vi "QPlus_Analyzer 3.0.vi"() -> ()   [LabVIEW 2017]
uses:
  <vilib>/express/express shared/transition.llb/Dynamic To Waveform Array.vi
  <vilib>/express/express signal manip/GetorSetDDTAttributes/Set DDT Attributes/SetT0.vi
  <vilib>/express/express shared/transition.llb/Waveform Array To Dynamic.vi
  <vilib>/express/express signal manip/GetorSetDDTAttributes/Set DDT Attributes/Set DDT Properties.xnode
  <instrlib>/Stanford Research 830/Stanford Research 830.lvlib
  <instrlib>/Agilent 3352X Series/Agilent 3352X Series.lvlib
panel:
  out "Resonance Frequency":dbl
  out "Y Signal":cluster{"Y":dbl[], "Y":dbl[]}[](graph)
  out "X Signal":cluster{"Y":dbl[], "Y":dbl[]}[](graph)
  in  "Reference name":refnum<visa-resource-name>
  in  "VISA resource name":refnum<visa-resource-name>
  in  "Sensitivity (26: 1 V/uA)":i8(ring)=20 items=["Auto Gain"=-1, "2 nV/fA"=0, "5 nV/fA"=1, "10 nV/fA"=2, "20 nV/fA"=3, "50 nV/fA"=4, "100 nV/fA"=5, "200 nV/fA"=6, "500 nV/fA"=7, "1 uV/pA"=8, "2 uV/pA"=9, "5 uV/pA"=10, "10 uV/pA"=11, "20 uV/pA"=12, "50 uV/pA"=13, "100 uV/pA"=14, "200 uV/pA"=15, "500 uV/pA"=16, "1 mV/nA"=17, "2 mV/nA"=18, "5 mV/nA"=19, "10 mV/nA"=20, "20 mV/nA"=21, "50 mV/nA"=22, "100 mV/nA"=23, "200 mV/nA"=24, "500 mV/mA"=25, "1 V/uA"=26]
  in  "Time Constant (6: 10ms)":u16(ring)=6 items=["10 us", "30 us", "100 us", "300 us", "1 ms", "3 ms", "10 ms", "30 ms", "100 ms", "300 ms", "1 s", "3 s", "10 s", "30 s", "100 s", "300 s", "1 ks", "3 ks", "10 ks", "30 ks"]
  in  "Save File Name":path=path "C:/Users/transport/Desktop/qPlus Tip Test/Data" caption="Filename"
  in  "Time Between Points (sec)":dbl=0.05 format="%#_1f"
  in  "Sine Output Amplitude (1 V)":dbl=0.1
  in  "Starting Frequency (Hz)":dbl=29000.0
  in  "Final Frequency (Hz)":dbl=32000.0
  in  "Step Size (Hz)":dbl=10.0
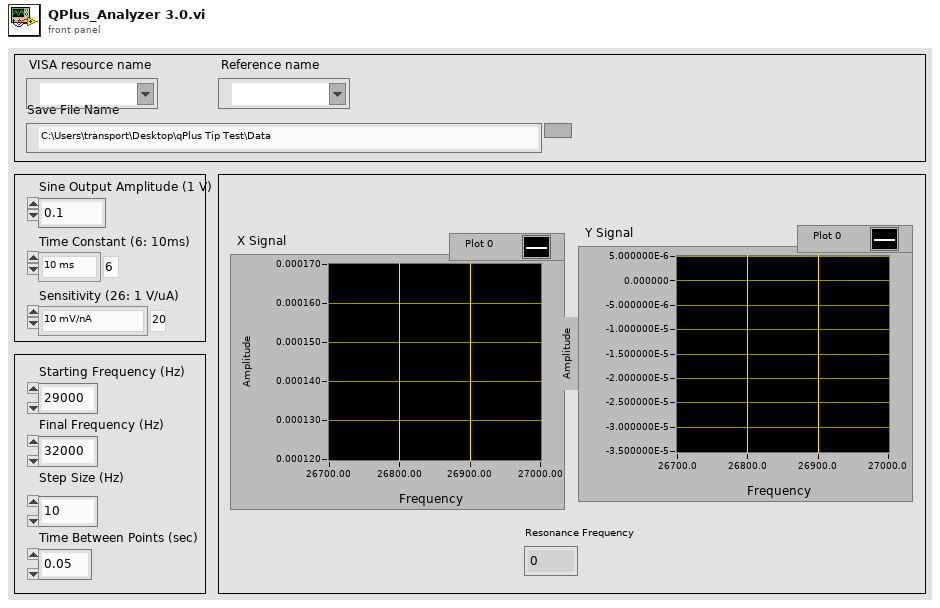
[diagram p1: front panel]
types:
  T1 = cluster{"X-Value":dbl, "Y-Value":dbl, "R-Value":dbl, "Theta-Value":dbl, "Aux In 1 Value":dbl, "Aux In 2 Value":dbl, "Aux In 3 Value":dbl, "Aux In 4 Value":dbl, "Reference Frequency":dbl, "Channel 1 Display":dbl, "Channel 2 Display":dbl}
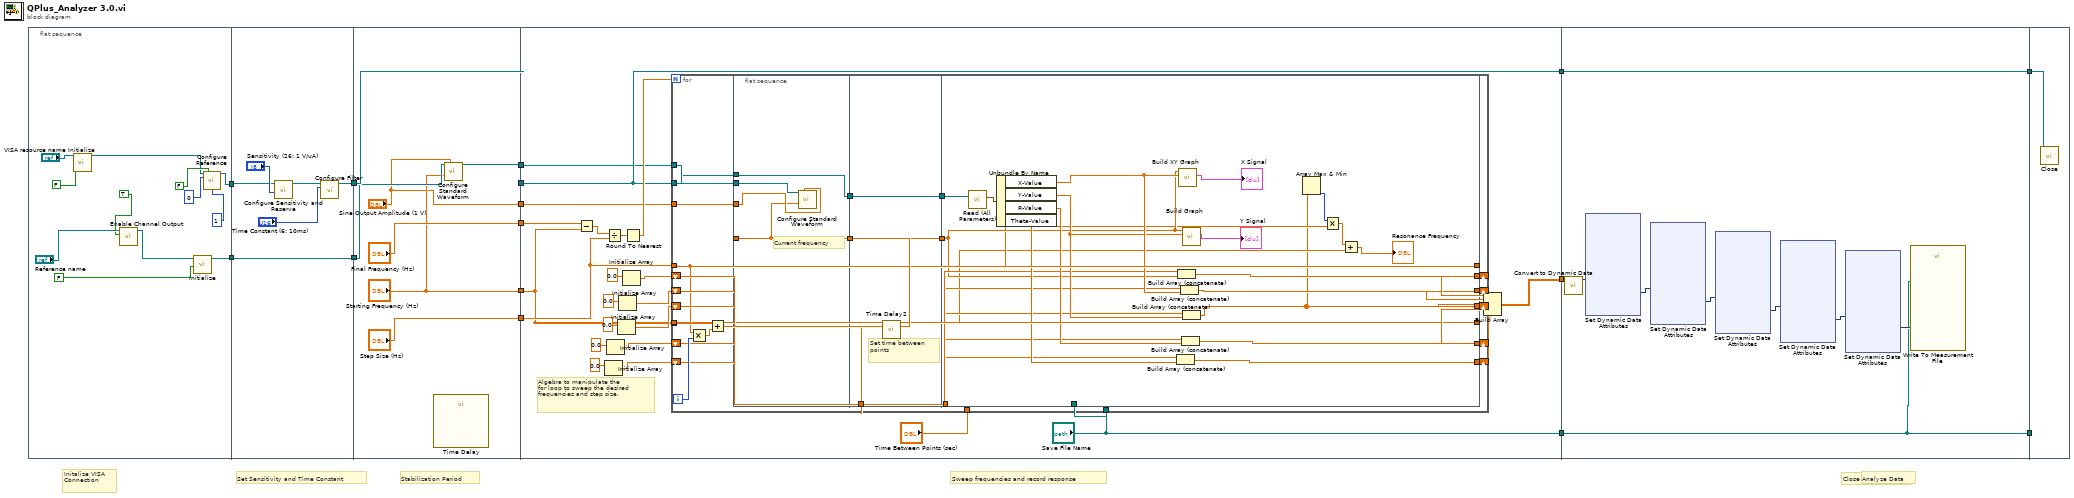
[diagram p0: block diagram]
diagram:
  # "Stabilization Period"
  # "Analyze Data"
  # "Close connection"
  # "Sweep frequencies and record response"
  # "Set Sensitivity and Time Constant"
  # "Initalize VISA\nConnection"
  n1 = flat-sequence {
    tunnel: [w23] -> w15
    tunnel: [w24] -> w7
    tunnel: [w30] -> w14
    tunnel: w15 -> [w29]
    tunnel: [w28] -> w8
    tunnel: w7 -> [w28]
    tunnel: w14 -> [w38]
    tunnel: [w38] -> w13
    tunnel: ["Starting Frequency (Hz)"] -> w12
    tunnel: ["Final Frequency (Hz)"] -> w11
    tunnel: ["Step Size (Hz)"] -> w10
    tunnel: ["Sine Output Amplitude (1 V)"] -> w9
    tunnel: w8 -> [w36]
    tunnel: [w37] -> w6
    tunnel: w13 -> [w64]
    tunnel: [w64] -> w5
    tunnel: ["Save File Name"] -> w3
    tunnel: w12 -> [w41]
    tunnel: w11 -> [w62]
    tunnel: w10 -> [w61]
    tunnel: w9 -> [w60]
    tunnel: w6 -> [w59]
    tunnel: [w42] -> w1
    tunnel: w5 -> [w132]
    tunnel: [w132] -> w4
    tunnel: w3 -> [w124]
    tunnel: [w124] -> w2
    tunnel: w1 -> [w125]
    tunnel: w4 -> [w203]
    tunnel: w2 -> [_]
    frame #0 {
      n2 = call <instrlib>:"Initialize.vi"("Reset (True)"=FALSE, "VISA resource name"="VISA resource name") -> ("VISA resource name out"=w16:refnum<visa-resource-name>)  [unwired: 8 in, 1 out]
      n3 = call <instrlib>:"Enable Channel Output.vi"("Enable Output (T: Enable)"=TRUE, "VISA resource name"="Reference name") -> ("VISA resource name out"=w18:refnum<visa-resource-name>)  [unwired: 8 in, 1 out]
      n4 = call <instrlib>:"Initialize.vi"("Reset (Enable)"=FALSE, "VISA resource name"=w18) -> ("VISA resource name out"=w24:refnum<visa-resource-name>)  [unwired: 8 in, 1 out]
      n5 = call "Configure Reference.vi"("VISA resource name"=w16, "Auto Phase (T: Enabled)"=FALSE, "Reference Source (1: Internal)"=0, "External Reference Trigger (0: Sine Zero Crossing)"=1) -> ("VISA resource name out"=w23:refnum<visa-resource-name>)  [unwired: 10 in, 1 out]
    }
    frame #1 {
      n6 = call <instrlib>:"Configure Sensitivity and Reserve.vi"("Sensitivity (-1: Auto gain)"="Sensitivity (26: 1 V/uA)", "VISA resource name"=w29) -> ("VISA resource name out"=w32:refnum<visa-resource-name>)  [unwired: 8 in, 1 out]
      n7 = call <instrlib>:"Configure Filter.vi"("Time Constant (8: 100ms)"="Time Constant (6: 10ms)", "VISA resource name"=w32) -> ("VISA resource name out"=w30:refnum<visa-resource-name>)  [unwired: 8 in, 1 out]
    }
    frame #2 {
      n8 = call "Time Delay"() -> ()  [unwired: 11 in, 1 out]
      n9 = call <instrlib>:"Configure Standard Waveform.vi"("VISA resource name"=w36, "Amplitude (0.1 Vpp)"="Sine Output Amplitude (1 V)", "Frequency/Sample Rate/Bandwidth (1000 Hz)"="Starting Frequency (Hz)") -> ("VISA resource name out"=w37:refnum<visa-resource-name>)  [unwired: 11 in, 1 out]
    }
    frame #3 {
      # "Algebra to manipulate the\nfor loop to sweep the desired\nfrequencies and step size."
      n10 = Subtract(x=w62, y=w41) -> (x-y=w67:dbl)
      n11 = Initialize Array(0.0 ("element")) -> (w43:dbl[])  [unwired: 1 in]
      n12 = Divide(x=w67, y=w61) -> (x/y=w66:dbl)
      n13 = Initialize Array(0.0 ("element")) -> (w44:dbl[])  [unwired: 1 in]
      n14 = Initialize Array(0.0 ("element")) -> (w45:dbl[])  [unwired: 1 in]
      n15 = Initialize Array(0.0 ("element")) -> (w46:dbl[])  [unwired: 1 in]
      n16 = Initialize Array(0.0 ("element")) -> (w47:dbl[])  [unwired: 1 in]
      n17 = Round To Nearest(number=w66) -> (nearest integer value=w65:dbl)
      n18 = for {
        N: w65 -> [_]
        tunnel: w61 -> [w69]
        tunnel: w41 -> [w90]
        tunnel: w64 -> [w81]
        tunnel: "Time Between Points (sec)" -> [w83]
        tunnel: "Save File Name" -> [w88]
        tunnel: w60 -> [w87]
        tunnel: w59 -> [w82]
        shift-right: [w79] -> w54
        shift-left: w46 -> [w74]
        shift-right: [w78] -> w55
        shift-left: w45 -> [w73]
        shift-right: [w70] -> w58
        shift-left: w47 -> [w75]
        shift-right: [w76] -> w56
        shift-left: w43 -> [w71]
        shift-right: [w77] -> w57
        shift-left: w44 -> [w72]
        tunnel: w41 -> [w68]
        i -> [w92]
        n19 = Multiply(x=w69, y=w92) -> (x*y=w91:dbl)
        n20 = Add(x=w90, y=w91) -> (x+y=w89:dbl)
        n21 = flat-sequence {
          tunnel: [w93] -> w85
          tunnel: w89 -> [w93]
          tunnel: w87 -> [w95]
          tunnel: w82 -> [w94]
          tunnel: w81 -> [w96]
          tunnel: [w96] -> w80
          tunnel: [w99] -> w86
          tunnel: w85 -> [w98]
          tunnel: [w98] -> w84
          tunnel: w83 -> [w97]
          tunnel: w80 -> [w99]
          tunnel: w86 -> [w121]
          tunnel: w84 -> [w107]
          tunnel: w88 -> [_]
          tunnel: [w120] -> w79
          tunnel: [w100] -> w78
          tunnel: [w115] -> w70
          tunnel: [w114] -> w77
          tunnel: [w113] -> w76
          tunnel: w75 -> [w112]
          tunnel: w74 -> [w111]
          tunnel: w73 -> [w110]
          tunnel: w72 -> [w109]
          tunnel: w71 -> [w108]
          tunnel: w69 -> [w105]
          tunnel: w68 -> [w103]
          frame #0 {
            # "Current frequency"
            n22 = call <instrlib>:"Configure Standard Waveform.vi"("VISA resource name"=w94, "Amplitude (0.1 Vpp)"=w95, "Frequency/Sample Rate/Bandwidth (1000 Hz)"=w93) -> ()  [unwired: 11 in, 2 out]
          }
          frame #1 {
            # "Set time between\npoints"
            n23 = call "Time Delay2"("Delay Time (s)"=w97) -> ()  [unwired: 10 in, 1 out]
          }
          frame #2 {
            n24 = call <instrlib>:"Read (All Parameters).vi"("VISA resource name"=w121) -> ("Parameter Values"=w122:T1)  [unwired: 8 in, 2 out]
            n25 = Unbundle By Name(w122) -> ("X-Value"=w119:dbl, "Y-Value"=w118:dbl, "R-Value"=w117:dbl, "Theta-Value"=w116:dbl)
            n26 = Build Array (concatenate)(w108, w116) -> (w113:dbl[])
            n27 = Build Array (concatenate)(w112, w107) -> (w115:dbl[])
            n28 = call "Build XY Graph"("Y Input"=w119, "X Input"=w107) -> ("XY Graph"=→"X Signal":cluster{"Y":dbl[], "Y":dbl[]}[])  [unwired: 3 in, 6 out]
            n29 = Build Array (concatenate)(w111, w119) -> (w120:dbl[])
            n30 = Build Array (concatenate)(w109, w117) -> (w114:dbl[])
            n31 = call "Build Graph"("Y Input"=w118, "X Input"=w107) -> ("XY Graph"=→"Y Signal":cluster{"Y":dbl[], "Y":dbl[]}[])  [unwired: 3 in, 6 out]
            n32 = Build Array (concatenate)(w110, w118) -> (w100:dbl[])
            n33 = Array Max & Min(array=w100) -> (min index (indices)=w101:i32)  [unwired: 3 out]
            n34 = Multiply(x=w101, y=w105) -> (x*y=w104:dbl)
            n35 = Add(x=w104, y=w103) -> (x+y=→"Resonance Frequency":dbl)
          }
        }
      }
      n36 = Build Array(w58, w54, w55, w57, w56) -> (w42:dbl[][])
    }
    frame #4 {
      n37 = call "Convert to Dynamic Data"("2D Array"=w125) -> ("Dynamic Data Type"=w131:dynamicdata)  [unwired: 3 in]
      n38 = xnode "Set Dynamic Data Attributes"("Signals In"=w131) -> ("Signals Out"=w126:dynamicdata)  [unwired: 3 in, 1 out]
      n39 = xnode "Set Dynamic Data Attributes"("Signals In"=w126) -> ("Signals Out"=w127:dynamicdata)  [unwired: 3 in, 1 out]
      n40 = xnode "Set Dynamic Data Attributes"("Signals In"=w127) -> ("Signals Out"=w128:dynamicdata)  [unwired: 3 in, 1 out]
      n41 = xnode "Set Dynamic Data Attributes"("Signals In"=w128) -> ("Signals Out"=w129:dynamicdata)  [unwired: 3 in, 1 out]
      n42 = xnode "Set Dynamic Data Attributes"("Signals In"=w129) -> ("Signals Out"=w130:dynamicdata)  [unwired: 3 in, 1 out]
      n43 = call "Write To Measurement File"("Signals"=w130, "Filename"=w124) -> ()  [unwired: 15 in, 3 out]
    }
    frame #5 {
      n44 = call <instrlib>:"Close.vi"("VISA resource name"=w203) -> ()  [unwired: 10 in, 1 out]
    }
  }
